vi "7HP_Clone.vi"(0 "Single 7HP":T1) -> (1 "Serial number":u32, 2 "DAQ Error":errorcluster, 3 "All samples out":sgl[][](array[numeric]), 4 "Ch No":i16[](array[numeric]), 5 "Index":i32[](array[numeric]), 6 "Sampling Rate Hz":dbl)   [LabVIEW 2021]
doc: "Use this plug-in with the Nathan 7609 data acquisition system"
uses:
  Device ID port info.ctl
  ctls/7HP_Cmd (USB).ctl
  Globals/Meas_global.vi
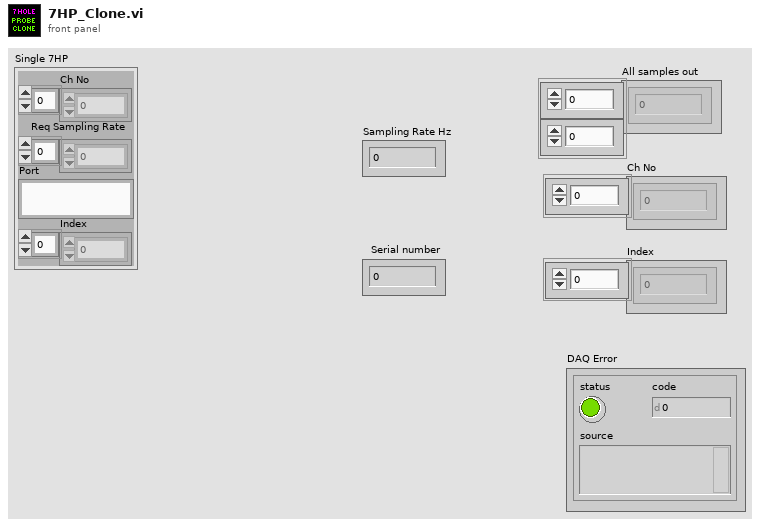
[diagram p1: front panel]
types:
  T1 = typedef "Device ID port info.ctl" = cluster{"Ch No":i16[], "Req Sampling Rate":dbl[], "Port":string, "Index":i32[]}
  T2 = typedef "Trigger_Mode.ctl" = enum16{"Free Running", "Start on Trigger", "Trigger Every Block", "Trigger Every Sample"}
  T3 = typedef "7HP_Cmd (USB).ctl" = string
  T4 = typedef "Rendezvous RefNum" = refnum<k1>
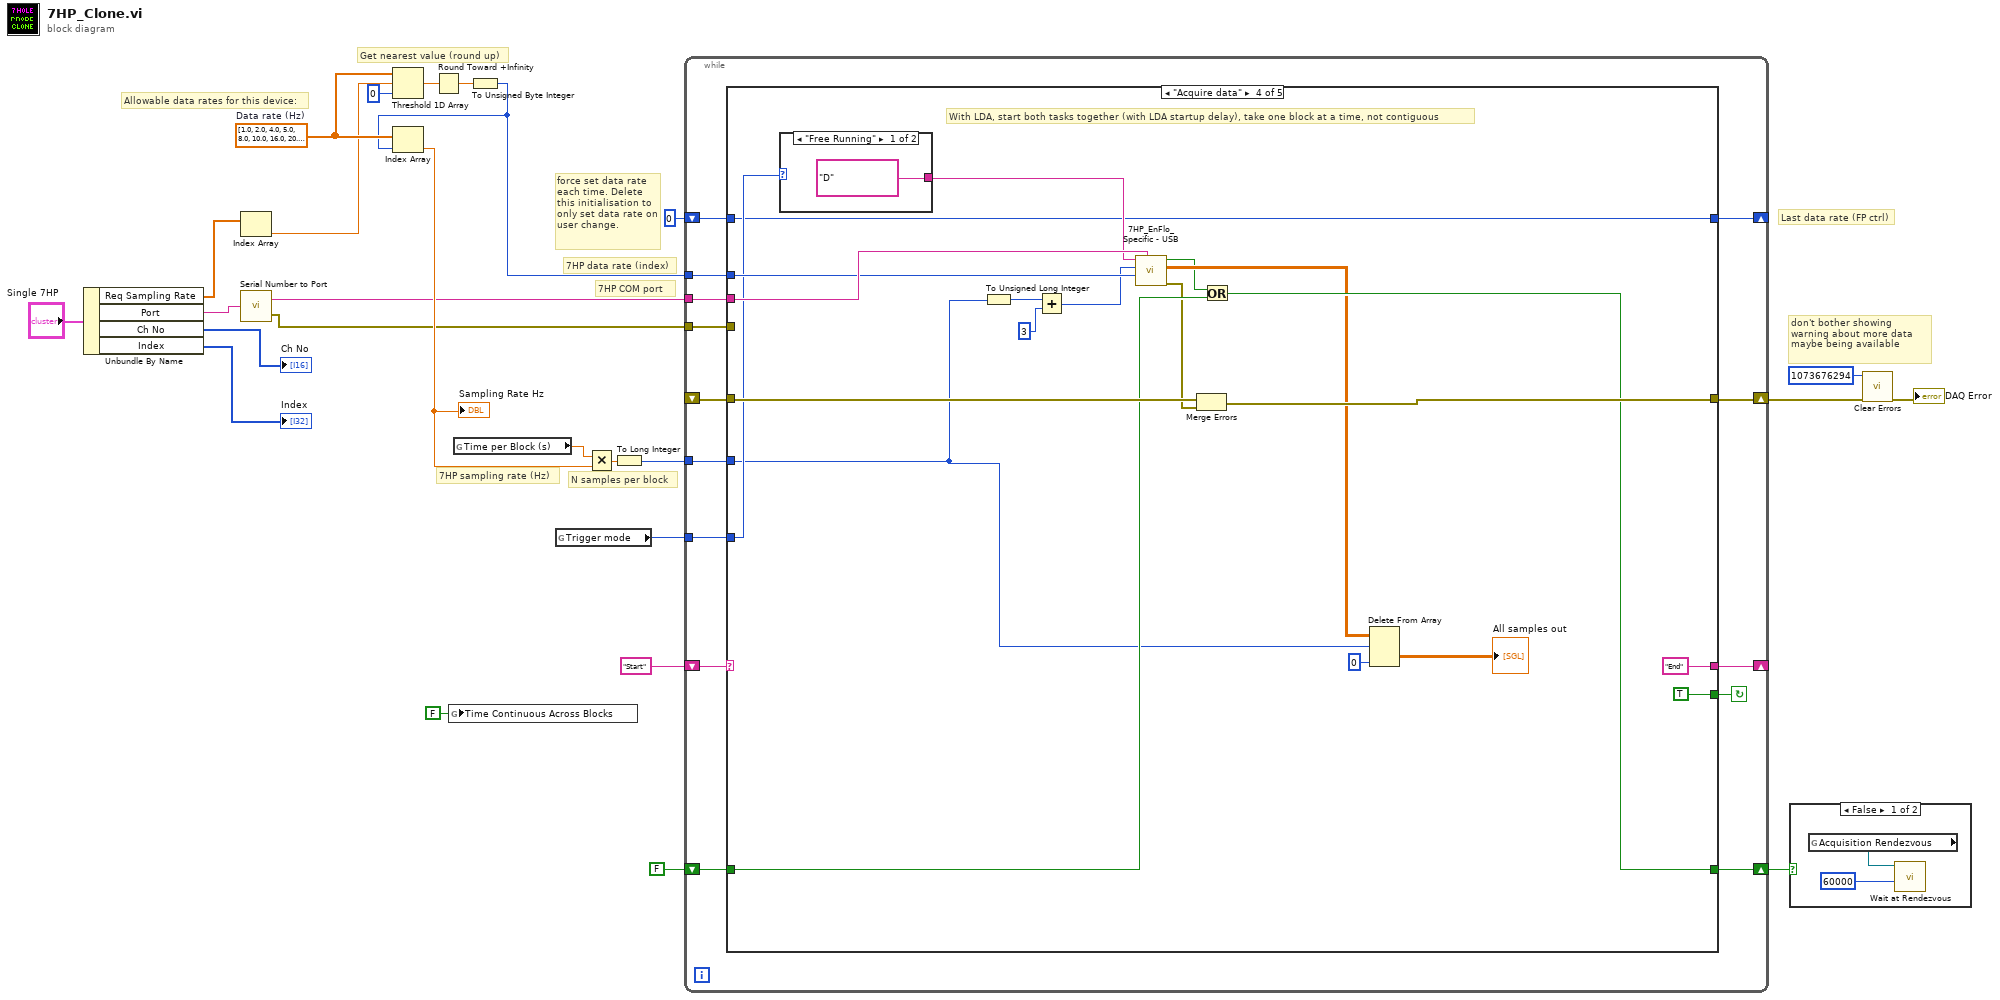
[diagram p0: block diagram]
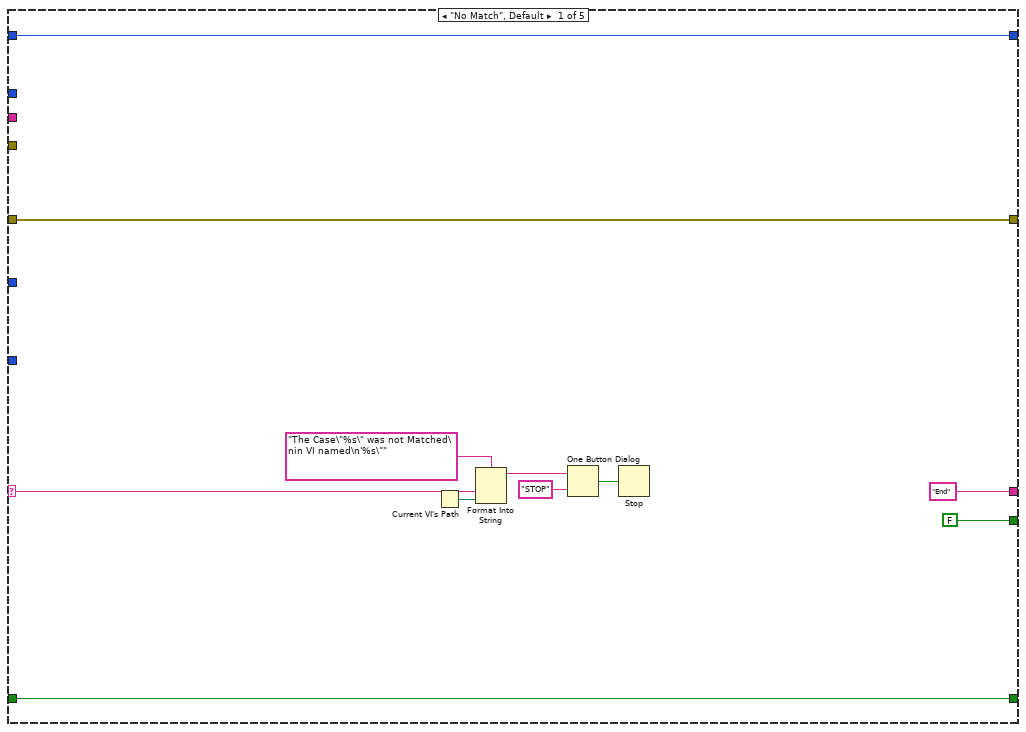
[diagram p3: hidden frame]
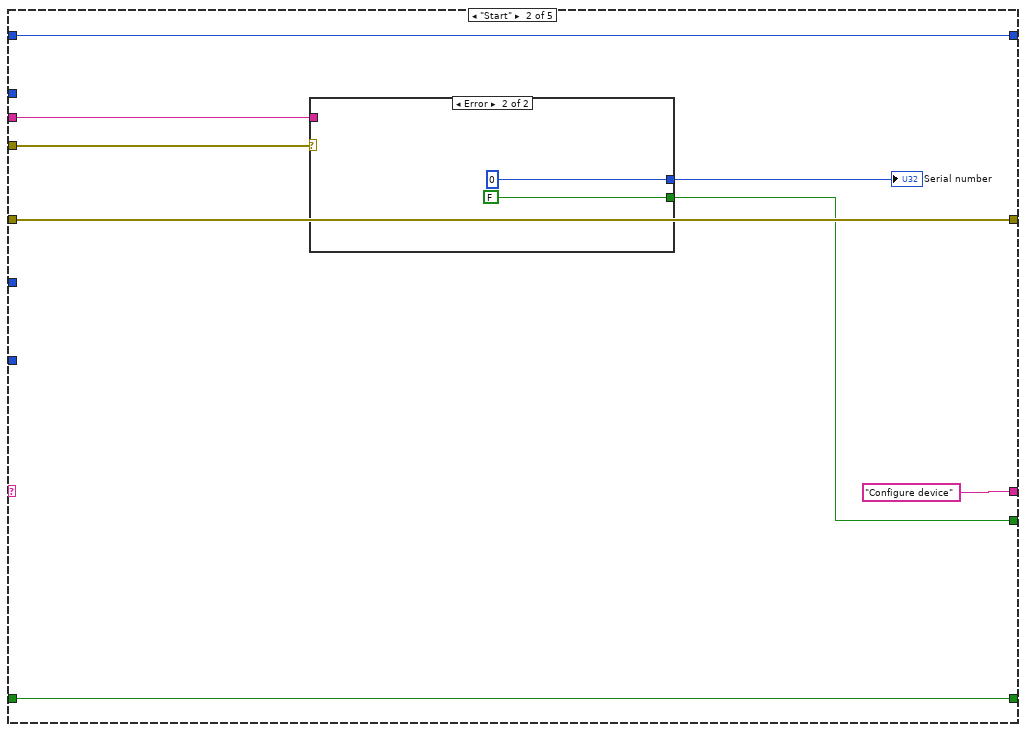
[diagram p4: hidden frame]
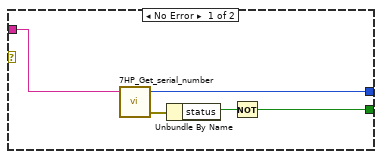
[diagram p5: hidden frame]
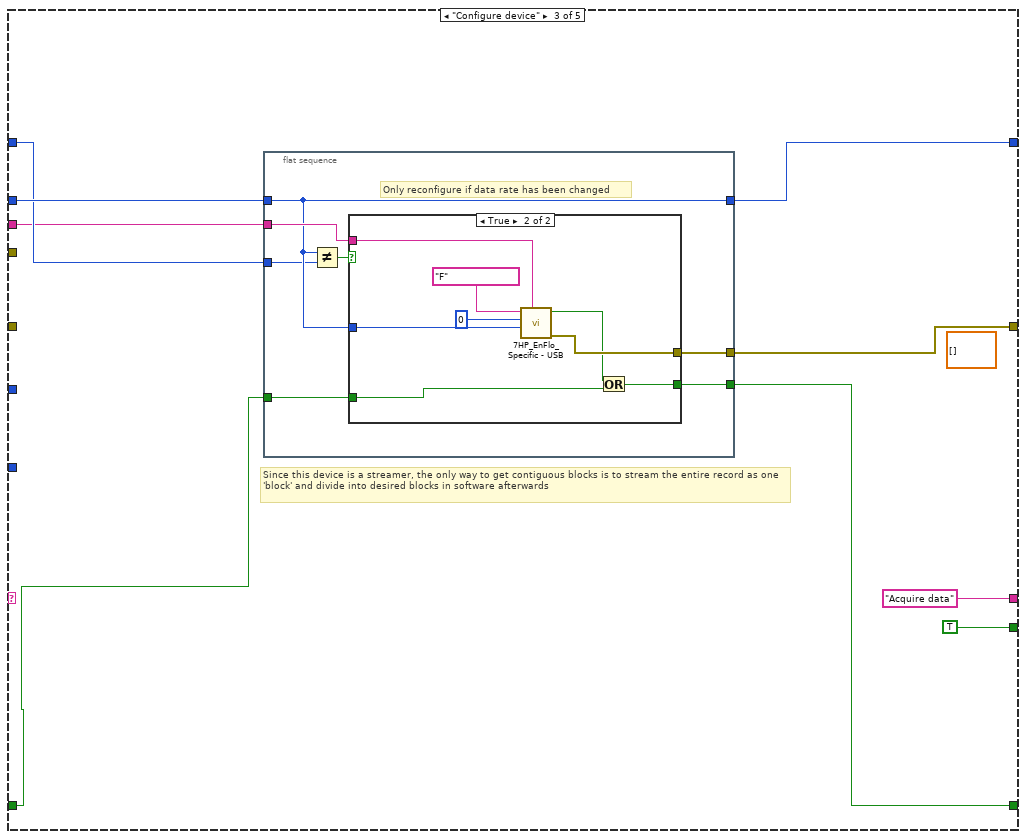
[diagram p6: hidden frame]
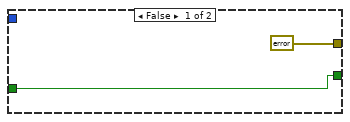
[diagram p7: hidden frame]
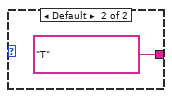
[diagram p8: hidden frame]
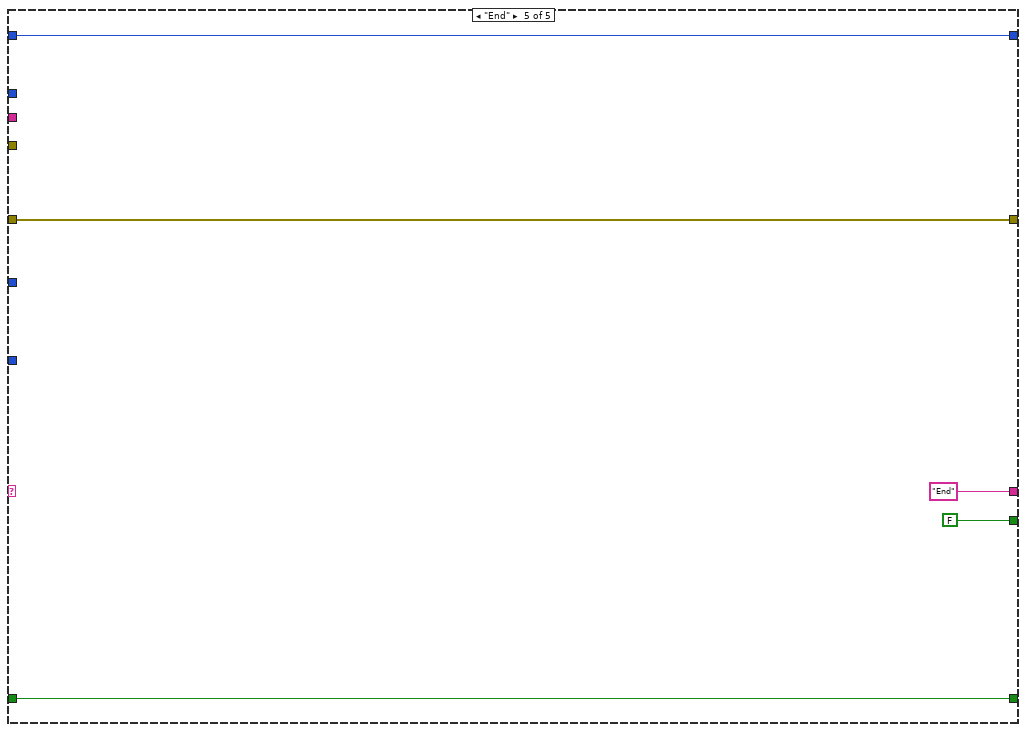
[diagram p9: hidden frame]
diagram:
  w18 = dbl[] [1.0, 2.0, 4.0, 5.0, 8.0, 10.0, 16.0, 20.0, 25.0, 32.0, 40.0, 50.0, 64.0, 80.0, 100.0, 125.0, 160.0, 200.0, 250.0, 320.0, 400.0, 500.0, 625.0, 800.0, 1000.0]  # Data rate (Hz)
  # "N samples per block"
  # "7HP sampling rate (Hz)"
  # "7HP COM port"
  # "7HP data rate (index)"
  # "Allowable data rates for this device:"
  # "Get nearest value (round up)"
  # "force set data rate each time. Delete this initialisation to only set data rate on user change."
  # "Last data rate (FP ctrl)"
  # "don't bother showing warning about more data maybe being available"
  n1 = Unbundle By Name("Single 7HP") -> ("Req Sampling Rate"=w10:dbl[], "Port"=w4:string, "Ch No"=→"Ch No":i16[], "Index"=→"Index":i32[])
  n2 = Index Array(array=w10) -> (element=w9:dbl)  [unwired: 1 in]
  n3 = call "Serial Number to Port.vi"("Port In"=w4) -> ("Port Out"=w6:string, "error out"=w5:errorcluster)
  n4 = Threshold 1D Array(1:0 ("start index (0)"), 2:w9, 3:w18) -> (0:w19:dbl)
  n5 = Round Toward +Infinity(x=w19) -> (ceil(x): smallest int >= x=w17:dbl)
  n6 = global write "Meas_global.vi" "Time Continuous Across Blocks"(FALSE ("Time Continuous Across Blocks")) -> ()
  n7 = global read "Meas_global.vi" "Time per Block (s)"() -> (w16:dbl)
  n8 = To Unsigned Byte Integer(number=w17) -> (unsigned 8bit integer=w12:u8)
  n9 = Index Array(array=w18, index=w12) -> (element=w13:dbl)
  "Sampling Rate Hz" <- w13
  n10 = global read "Meas_global.vi" "Trigger mode"() -> (w25:T2)
  n11 = Multiply(x=w16, y=w13) -> (x*y=w15:dbl)
  n12 = To Long Integer(number=w15) -> (32bit integer=w14:i32)
  n13 = while {
    shift-left: "Start" -> [w40]
    shift-right: [w34] -> _
    tunnel: w14 -> [w39]
    tunnel: w25 -> [w37]
    shift-right: [w35] -> w22
    shift-left: _ -> [w36]
    tunnel: w6 -> [w33]
    tunnel: w12 -> [w32]
    shift-right: [w31] -> _
    shift-left: u8 0 ("Pressure data rate (Hz)") -> [w30]
    tunnel: w5 -> [w29]
    shift-right: [w28] -> w2
    shift-left: FALSE -> [w27]
    stop <- w38 continue-if-true
    n14 = case shown="\"Acquire data\"" w40 {
      selector: w40 -> [w44 _ _ _ _]
      tunnel: ["End" "Configure device" ("f") "Acquire data" ("f") "End" "End" ("f")] -> w34
      tunnel: w39 -> [_ _ _ w96 _]
      tunnel: [FALSE w53 TRUE TRUE FALSE] -> w38
      tunnel: w37 -> [_ _ _ w105 _]
      tunnel: w36 -> [w43 w59 _ w110 w117]
      tunnel: [w43 w59 w74 w109 w117] -> w35
      tunnel: w33 -> [_ w55 w69 w108 _]
      tunnel: w32 -> [_ _ w72 w107 _]
      tunnel: [w42 w57 w71 w103 w116] -> w31
      tunnel: w30 -> [w42 w57 w70 w103 w116]
      tunnel: w29 -> [_ w56 _ _ _]
      tunnel: [w41 w52 w67 w101 w115] -> w28
      tunnel: w27 -> [w41 w52 w68 w102 w115]
      frame "No Match", Default {
        n15 = Current VI's Path() -> (path=w47:path)
        n16 = Format Into String(format string="The Case\"%s\" was not Matched\nin VI named\n'%s\"" ("Format String"), w44, w47) -> (resulting string=w50:string)  [unwired: 2 in, 1 out]
        n17 = One Button Dialog(message=w50, button name ("OK")="STOP") -> (true=w48:bool)
        n18 = Stop(stop? (T)=w48) -> ()
      }
      frame "Start" {
        n19 = case shown="Error" w56 {
          tunnel: w55 -> [w64 _]
          tunnel: [w63 u32 0 ("Serial number")] -> w54
          tunnel: [w60 FALSE] -> w53
          frame No Error {
            n20 = call "7HP_Get_serial_number.vi"("Port"=w64) -> ("Error Out"=w62:errorcluster, "Serial number"=w63:u32)  [unwired: 3 in]
            n21 = Unbundle By Name(w62) -> ("status"=w61:bool)
            n22 = Not(x=w61) -> (.not. x?=w60:bool)
          }
          frame Error {
          }
        }
        "Serial number" <- w54
      }
      frame "Configure device" {
        (unwired) sgl[][] [] ("Channel volts")
        # "Since this device is a streamer, the only way to get contiguous blocks is to stream the entire record as one 'block' and divide into desired blocks in software afterwards"
        n23 = flat-sequence {
          tunnel: [w82] -> w74
          tunnel: w69 -> [w81]
          tunnel: w72 -> [w79]
          tunnel: [w79] -> w71
          tunnel: w70 -> [w78]
          tunnel: w68 -> [w77]
          tunnel: [w76] -> w67
          frame #0 {
            # "Only reconfigure if data rate has been changed"
            n24 = Not Equal?(x=w79, y=w78) -> (x != y?=w80:bool)
            n25 = case shown="True" w80 {
              tunnel: [errorcluster {"status"=FALSE, "code"=0, "source"=""} ("error IO") w89] -> w82
              tunnel: w81 -> [_ w88]
              tunnel: w79 -> [_ w90]
              tunnel: w77 -> [w83 w86]
              tunnel: [w83 w85] -> w76
              frame False {
              }
              frame True {
                n26 = call "7HP_EnFlo_Specific - USB.vi"("COM port"=w88, "Set data rate (Hz)"=w90, "N samples"=u32 0, "Command"=T3 "F") -> ("Error"=w89:errorcluster, "Rendezvous out"=w87:bool)  [unwired: 4 in, 1 out]
                n27 = Or(x=w87, y=w86) -> (x .or. y?=w85:bool)
              }
            }
          }
        }
      }
      frame "Acquire data" {
        # "With LDA, start both tasks together (with LDA startup delay), take one block at a time, not contiguous"
        n28 = case shown="\"Free Running\"" w105 {
          tunnel: [T3 "D" ("Command") T3 "T" ("Command")] -> w106
          frame "Free Running" {
          }
          frame Default {
          }
        }
        n29 = To Unsigned Long Integer(number=w96) -> (unsigned 32bit integer=w95:u32)
        n30 = Add(x=w95, y=u32 3) -> (x+y=w93:u32)
        n31 = call "7HP_EnFlo_Specific - USB.vi"("COM port"=w108, "Set data rate (Hz)"=w107, "N samples"=w93, "Command"=w106) -> ("Error"=w100:errorcluster, "All samples out"=w99:sgl[][], "Rendezvous out"=w97:bool)  [unwired: 4 in]
        n32 = Merge Errors(w110, w100) -> (w109:errorcluster)
        n33 = Or(x=w97, y=w102) -> (x .or. y?=w101:bool)
        n34 = Delete From Array(array=w99, length=w96, index (col)=0 ("disabled index (col)")) -> (deleted portion=→"All samples out":sgl[][])  [unwired: 1 in, 1 out]
      }
      frame "End" {
      }
    }
  }
  n35 = case shown="False" w2 {
    frame False {
      n36 = global read "Meas_global.vi" "Acquisition Rendezvous"() -> (w121:T4)
      n37 = call <vilib>:"Wait at Rendezvous.vi"("ms timeout (-1)"=60000, "rendezvous"=w121) -> ()  [unwired: 3 in, 3 out]
    }
    frame True {
    }
  }
  n38 = call <vilib>:"Clear Errors.vi"("error in (no error)"=w22, "specific error code to clear (0: all)"=1073676294) -> ("error out"=→"DAQ Error":errorcluster)  [unwired: 4 in, 1 out]
